vi "Set Valve Pos Impl.vi"(8 "error in (no error)":errorcluster, 10 "Valve Pos":u16, 11 "Simulated Autosampler in":refnum<class "Simulated Autosampler.lvclass">) -> (0 "error out":errorcluster, 3 "Simulated Autosampler out":refnum<class "Simulated Autosampler.lvclass">)   [LabVIEW 2023, in "Simulated Autosampler.lvlib" / "Simulated Autosampler.lvclass"]
uses:
  Simulated Autosampler.lvclass
  Simulated Autosampler.lvclass/Simulated Autosampler.ctl
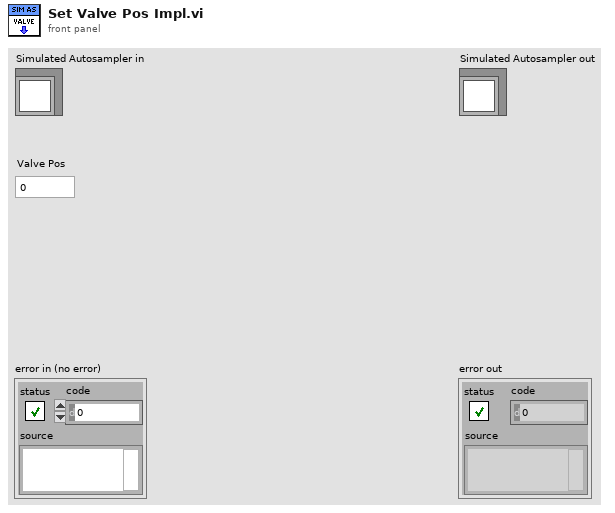
[diagram p1: front panel]
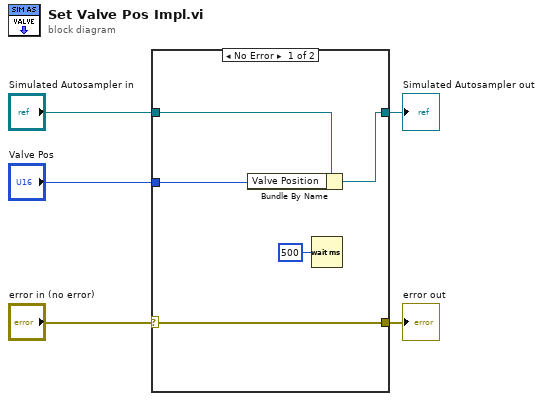
[diagram p0: block diagram]
diagram:
  n1 = case shown="No Error" "error in (no error)" {
    selector: "error in (no error)" -> [w10 w11]
    tunnel: [w10 w11] -> w4
    tunnel: "Simulated Autosampler in" -> [w8 w12]
    tunnel: [w7 w12] -> w2
    tunnel: "Valve Pos" -> [w9 _]
    frame No Error {
      n2 = Bundle By Name(cluster=w8, "Valve Position"=w9) -> (w7:refnum<class "Simulated Autosampler.lvclass">)
      n3 = Wait (ms)(milliseconds to wait=u32 500) -> ()  [unwired: 1 out]
    }
    frame Error {
    }
  }
  "error out" <- w4
  "Simulated Autosampler out" <- w2
